vi "Save Mov Dev config.vi"(7 "Montura":T2, 8 "error in (no error)":errorcluster, 9 "Datos Zaber":T3, 10 "Datos Bipolar/Unipolar":T4 {"Numero de lecturas" max=910098 step=1}, 11 "Refnum in":T1) -> (0 "error out":errorcluster, 3 "refnum out":T1)   [LabVIEW 2020]
uses:
  <vilib>/Utility/config.llb/NI_LVConfig.lvlib
  <vilib>/Utility/config.llb/Write Key (Boolean).vi
  <vilib>/Utility/config.llb/Write Key (U32).vi
  <vilib>/Utility/config.llb/Write Key (String).vi
  <vilib>/Utility/config.llb/Write Key (Double).vi
  <vilib>/Utility/config.llb/Config Data RefNum.ctl
  Type Definitions/parametros motores.ctl
  Type Definitions/Datos Zaber.ctl
  H:/Mi unidad/Departamento de Ingenieria/Investigadores/Gabriel Ramos/Proyecto Monturas v13/LV Source/Type Definitions/Tipos de montura.ctl
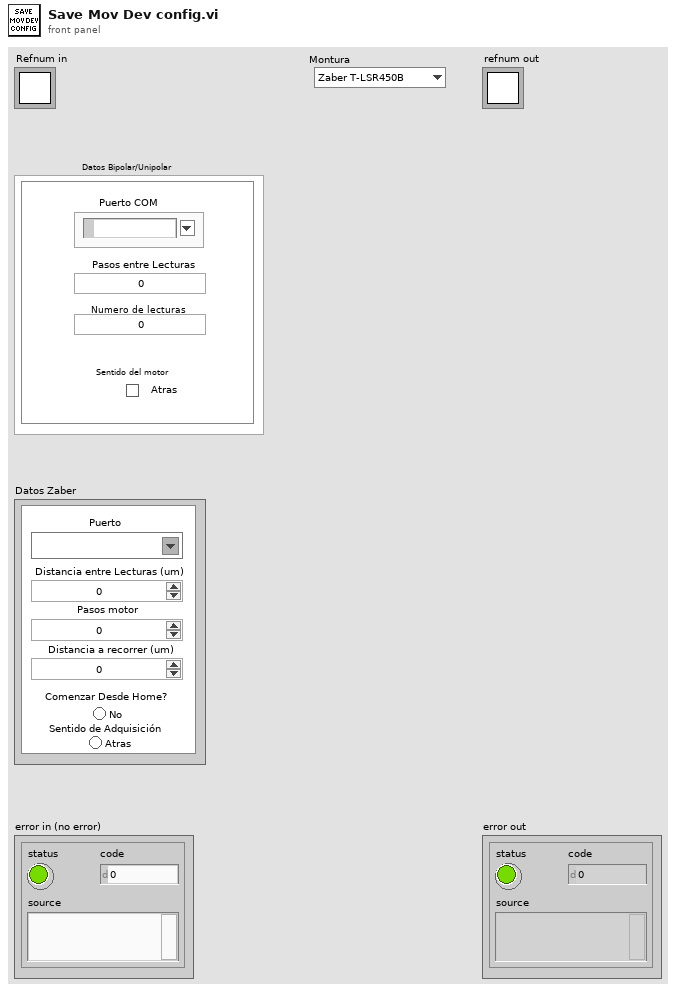
[diagram p1: front panel]
types:
  T1 = typedef "NI_LVConfig.lvlib/Config Data RefNum.ctl" = refnum<k1>
  T2 = typedef "Tipos de montura.ctl" = enum16{"Zaber T-LSR450B", "Zaber-T-LSR300B", "Zaber-T-LSRxxx", "Motor Bipolar", "Motor Unipolar"}
  T3 = typedef "Datos Zaber.ctl" = cluster{"Sentido de Adquisición":bool, "Comenzar Desde Home?":bool, "Distancia a recorrer (um)":dbl, "Pasos motor":i32, "Distancia entre Lecturas (um)":dbl, "Puerto":refnum<visa-resource-name>}
  T4 = typedef "parametros motores.ctl" = cluster{"Puerto COM":refnum<visa-resource-name>, "Pasos entre Lecturas":u16, "Numero de lecturas":u32, "Sentido del motor":bool}
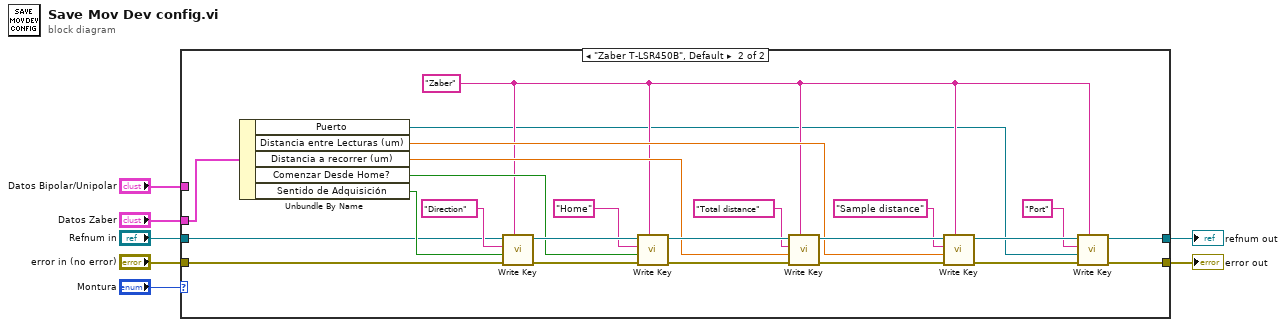
[diagram p0: block diagram]
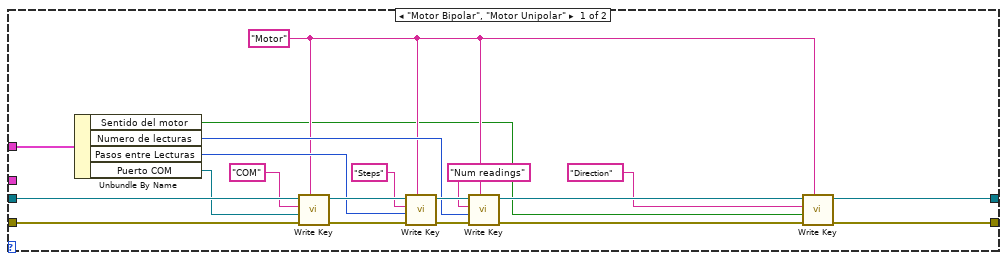
[diagram p2: hidden frame]
diagram:
  n1 = case shown="\"Zaber T-LSR450B\", Default" "Montura" {
    tunnel: "Datos Zaber" -> [_ w49]
    tunnel: "Datos Bipolar/Unipolar" -> [w24 _]
    tunnel: "Refnum in" -> [w26 w46]
    tunnel: "error in (no error)" -> [w27 w51]
    tunnel: [w13 w33] -> w2
    tunnel: [w11 w31] -> w1
    frame "Motor Bipolar", "Motor Unipolar" {
      w10 = "Motor" ("section")
      n2 = Unbundle By Name(w24) -> ("Sentido del motor"=w8:bool, "Numero de lecturas"=w15:u32, "Pasos entre Lecturas"=w18:u16, "Puerto COM"=w20:refnum<visa-resource-name>)
      n3 = call-poly <vilib>:"Write Key.vi"("section"=w10, "error in (no error)"=w27, "value"=w20, "key"="COM", "refnum"=w26) -> ("error out"=w25:errorcluster, "refnum out"=w22:T1)  [unwired: 4 in, 1 out]
      n4 = call-poly <vilib>:"Write Key.vi"("section"=w10, "error in (no error)"=w25, "value"=w18, "key"="Steps", "refnum"=w22) -> ("error out"=w23:errorcluster, "refnum out"=w17:T1)  [unwired: 4 in, 1 out]
      n5 = call-poly <vilib>:"Write Key.vi"("section"=w10, "error in (no error)"=w23, "value"=w15, "key"="Num readings", "refnum"=w17) -> ("error out"=w14:errorcluster, "refnum out"=w12:T1)  [unwired: 4 in, 1 out]
      n6 = call-poly <vilib>:"Write Key.vi"("section"=w10, "error in (no error)"=w14, "value"=w8, "key"="Direction", "refnum"=w12) -> ("error out"=w13:errorcluster, "refnum out"=w11:T1)  [unwired: 4 in, 1 out]
    }
    frame "Zaber T-LSR450B", Default {
      w30 = "Zaber" ("section")
      n7 = Unbundle By Name(w49) -> ("Puerto"=w28:refnum<visa-resource-name>, "Distancia entre Lecturas (um)"=w34:dbl, "Distancia a recorrer (um)"=w39:dbl, "Comenzar Desde Home?"=w43:bool, "Sentido de Adquisición"=w47:bool)
      n8 = call-poly <vilib>:"Write Key.vi"("section"=w30, "error in (no error)"=w51, "value"=w47, "key"="Direction", "refnum"=w46) -> ("error out"=w50:errorcluster, "refnum out"=w44:T1)  [unwired: 4 in, 1 out]
      n9 = call-poly <vilib>:"Write Key.vi"("section"=w30, "error in (no error)"=w50, "value"=w43, "key"="Home", "refnum"=w44) -> ("error out"=w45:errorcluster, "refnum out"=w40:T1)  [unwired: 4 in, 1 out]
      n10 = call-poly <vilib>:"Write Key.vi"("section"=w30, "error in (no error)"=w45, "value"=w39, "key"="Total distance", "refnum"=w40) -> ("error out"=w41:errorcluster, "refnum out"=w36:T1)  [unwired: 4 in, 1 out]
      n11 = call-poly <vilib>:"Write Key.vi"("section"=w30, "error in (no error)"=w41, "value"=w34, "key"="Sample distance", "refnum"=w36) -> ("error out"=w37:errorcluster, "refnum out"=w32:T1)  [unwired: 4 in, 1 out]
      n12 = call-poly <vilib>:"Write Key.vi"("section"=w30, "error in (no error)"=w37, "value"=w28, "key"="Port", "refnum"=w32) -> ("error out"=w33:errorcluster, "refnum out"=w31:T1)  [unwired: 4 in, 1 out]
    }
  }
  "error out" <- w2
  "refnum out" <- w1
